vi "Set Speed From State.vi"(11 "Public Methods:State":T1) -> (3 "Output":dbl)   [LabVIEW 2019, in "Cargo.lvlib" / "Cargo.lvclass"]
doc: "The VI gets the Cargo State and then depending on the state outputs cargo speed. The range is between -1 to 1."
uses:
  Cargo.lvclass
  Controls/Cargo States.ctl
  <vilib>/Rock Robotics/Network Tables/NT Read String.vi
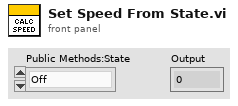
[diagram p1: front panel]
types:
  T1 = typedef "Cargo.lvlib/Cargo.lvclass/Cargo States.ctl" = enum16{"Off", "Intake Full", "Intake Idle", "Output Full"}
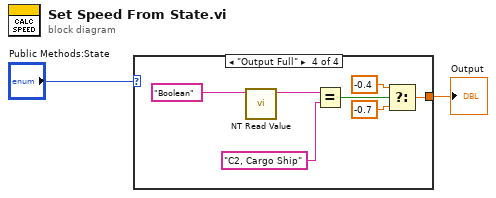
[diagram p0: block diagram]
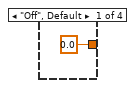
[diagram p2: hidden frame]
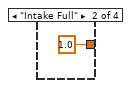
[diagram p3: hidden frame]
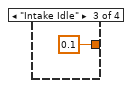
[diagram p4: hidden frame]
diagram:
  n1 = case shown="\"Output Full\"" "Public Methods:State" {
    tunnel: [0.0 ("Output") 1.0 ("Output") 0.1 ("Output") w6] -> w2
    frame "Off", Default {
    }
    frame "Intake Full" {
    }
    frame "Intake Idle" {
    }
    frame "Output Full" {
      n2 = call-poly <vilib>:"NT Read Value.vi"("Name"="Boolean" ("Elevator Position")) -> ("String"=w10:string)  [unwired: 9 in, 1 out]
      n3 = Equal?(x=w10, y="C2, Cargo Ship") -> (x = y?=w12:bool)
      n4 = Select(t=-0.4, s=w12, f=-0.7 ("Output")) -> (s? t:f=w6:dbl)
    }
  }
  "Output" <- w2
